vi "Read Core.vi"(8 "error in (no error)":errorcluster, 9 "Timeout (1s)":dbl[unit]=1.0, 11 "PVConnection in":refnum<class "DSConnection.lvclass">) -> (0 "error out":errorcluster, 1 "timed out":bool, 2 "PV":refnum<class "PV.lvclass">, 3 "PVConnection out":refnum<class "DSConnection.lvclass">)   [LabVIEW 2015, in "CS++ProcessVariables.lvlib" / "DSConnection.lvclass"]
doc: "Read a process variable."
uses:
  DSConnection.lvclass
  ProcessVariable/PV.lvclass
  DSConnection.lvclass/DSConnection.ctl
  PVConnection/PVConnection.lvclass/PVConnection.ctl
  ProcessVariable/PV.lvclass/PV.ctl
  CS++BaseClasses/Base/CS++Base.lvclass/CS++Base.ctl
  ProcessVariable/Write Data.vi
  ProcessVariable/Write Error.vi
  ProcessVariable/Write Timestamp.vi
  ProcessVariable/Write status.vi
  ProcessVariable/Write Quality.vi
  PVConnection/PVConnection.lvclass
  Libraries/Utilities/CS++Utilities.lvlib
  CS++BaseClasses/Base/CS++Base.lvclass
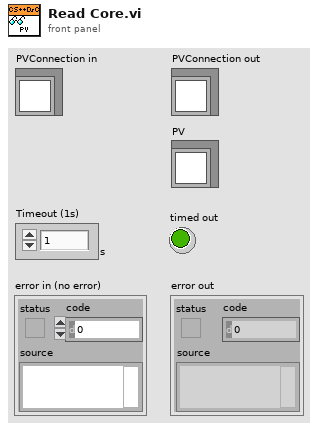
[diagram p1: front panel]
types:
  T1 = cluster{"Read Access":enum8{"Allowed", "Required", "None"}, "Write Access":enum8{"Allowed", "Required", "None"}}
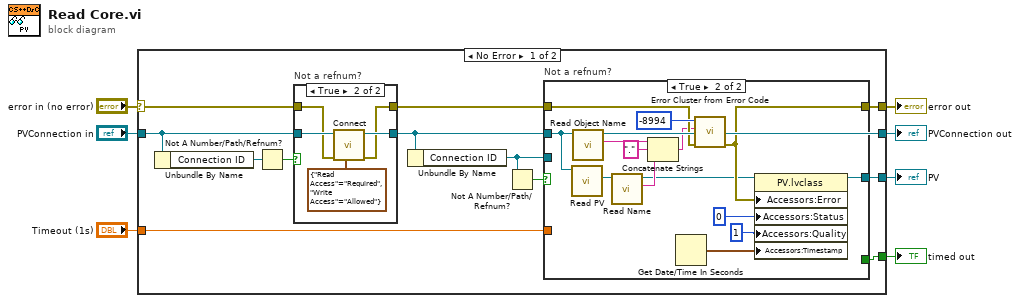
[diagram p0: block diagram]
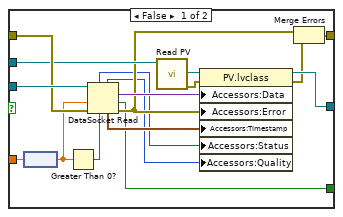
[diagram p3: hidden frame]
diagram:
  n1 = case shown="No Error" "error in (no error)" {
    selector: "error in (no error)" -> [w11 w58]
    tunnel: [w19 w58] -> w4
    tunnel: [w12 w59] -> w5
    tunnel: "PVConnection in" -> [w13 w59]
    tunnel: [w16 _] -> w3
    tunnel: "Timeout (1s)" -> [w9 _]
    tunnel: [w8 _] -> w1
    frame No Error {
      n2 = Unbundle By Name(w13) -> ("Connection ID"=w15:refnum<k13>)
      n3 = Not A Number/Path/Refnum?(number/path/refnum=w15) -> (NaN/Path/Refnum?=w14:bool)
      n4 = case "Not a refnum?" shown="True" w14 {
        tunnel: w13 -> [w20 w26]
        tunnel: [w20 w25] -> w12
        tunnel: w11 -> [w21 w24]
        tunnel: [w21 w23] -> w10
        frame False {
        }
        frame True {
          n5 = call "Connect.vi"("Access (R/W allowed)"=T1 {"Read Access"=enum."Required", "Write Access"=enum."Allowed"}, "Error In"=w24, "PVConnection in"=w26) -> ("Error Out"=w23:errorcluster, "PVConnection out"=w25:refnum<class "DSConnection.lvclass">)  [unwired: 7 in]
        }
      }
      n6 = Unbundle By Name(w12) -> ("Connection ID"=w17:refnum<k13>)
      n7 = Not A Number/Path/Refnum?(number/path/refnum=w17) -> (NaN/Path/Refnum?=w18:bool)
      n8 = case "Not a refnum?" shown="True" w18 {
        tunnel: w17 -> [w43 _]
        tunnel: w10 -> [w42 w56]
        tunnel: [w34 w54] -> w19
        tunnel: w12 -> [w41 w47]
        tunnel: [w38 w55] -> w16
        tunnel: w9 -> [w30 _]
        tunnel: [w29 _] -> w8
        frame False {
          n9 = node(w30) -> (w28:dbl)
          n10 = Greater Than 0?(x=w28) -> (x > 0?=w27:bool)
          n11 = DataSocket Read(6:w27, 8:w42, 9:w28, 11:w43) -> (0:w33:errorcluster, 1:w29:bool, 2:w40:variant, 4:w39:timestamp, 5:w31:u64, 7:w32:u32)  [unwired: 1 in, 1 out]
          n12 = call "Read PV.vi"("PVConnection in"=w41) -> ("error out"=w36:errorcluster, "PV"=w37:refnum<class "PV.lvclass">)  [unwired: 8 in, 1 out]
          n13 = property class="PV.lvclass"(reference=w37, error in=w36, "Accessors:Data"=w40, "Accessors:Error"=w33, "Accessors:Timestamp"=w39, "Accessors:Status"=w32, "Accessors:Quality"=w31) -> (reference out=w38:refnum<class "PV.lvclass">, error out=w35:errorcluster)
          n14 = Merge Errors(w33, w35) -> (w34:errorcluster)
        }
        frame True {
          n15 = call "Read PV.vi"("PVConnection in"=w47) -> ("PV"=w49:refnum<class "PV.lvclass">)  [unwired: 8 in, 2 out]
          n16 = call "Read Object Name.vi"("Base in"=w47) -> ("Object Name"=w45:string)  [unwired: 8 in, 2 out]
          n17 = call "Read Name.vi"("PV in"=w49) -> ("Name"=w50:string, "PV out"=w48:refnum<class "PV.lvclass">)  [unwired: 8 in, 1 out]
          n18 = Concatenate Strings(w45, "." ("string"), w50) -> (w46:string)
          n19 = Get Date/Time In Seconds() -> (seconds since 1Jan1904=w51:timestamp)
          n20 = call "Error Cluster from Error Code.vi"("Error In"=w56, "Error Message (\"\")"=w46, "Error Code (0)"=-8994 ("error code (0)")) -> ("Error Out"=w54:errorcluster)  [unwired: 8 in]
          n21 = property class="PV.lvclass"(reference=w48, "Accessors:Error"=w54, "Accessors:Status"=u32 0 ("status"), "Accessors:Quality"=u64 1 ("quality"), "Accessors:Timestamp"=w51) -> (reference out=w55:refnum<class "PV.lvclass">)  [unwired: 1 in, 1 out]
        }
      }
    }
    frame Error {
    }
  }
  "error out" <- w4
  "PVConnection out" <- w5
  "PV" <- w3
  "timed out" <- w1
